vi "testConfig.vi"(8 "error in (no error)":errorcluster) -> (0 "error out":errorcluster)   [LabVIEW 2018]
uses:
  src/Logger/Logger.lvclass
  src/Logger/Logger.lvclass/Logger.ctl
  <vilib>/addons/_JKI Toolkits/Caraya/classes/Assert/Assert Equal Value_Variant.vi
  <vilib>/addons/_JKI Toolkits/Caraya/classes/Assert/Assert True.vi
  <vilib>/addons/_JKI Toolkits/Caraya/classes/Test/Test.lvclass
  <vilib>/addons/_JKI Toolkits/Caraya/classes/Assert/Assert.lvclass
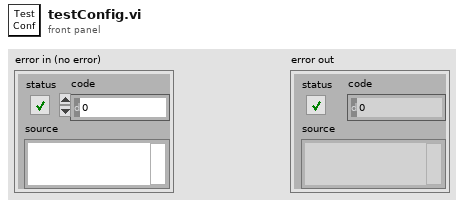
[diagram p1: front panel]
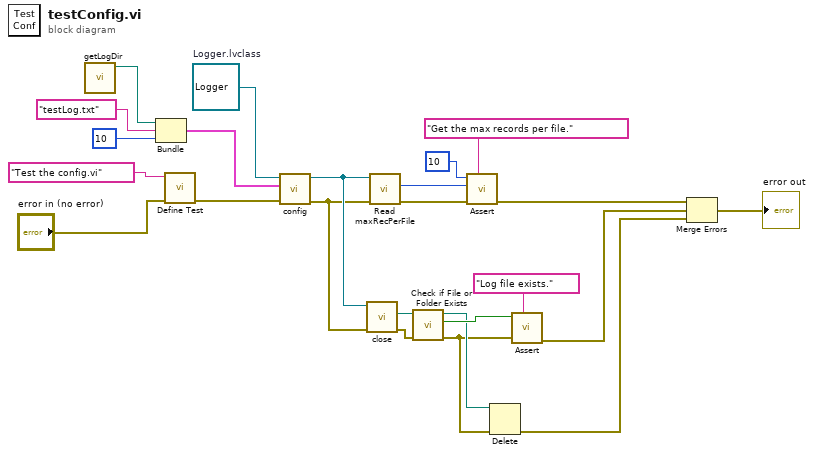
[diagram p0: block diagram]
diagram:
  w21 = refnum<class "Logger.lvclass"> refnum  # Logger.lvclass
  n1 = call "getLogDir.vi"() -> ("dirLog"=w20:path)  [unwired: 11 in]
  n2 = Bundle("dirLog"=w20, "testLog.txt", u32 10) -> (w17:cluster{"dirLog":path, string, u32})  [unwired: 1 in]
  n3 = call <vilib>:"Define Test.vi"("error in (no error)"="error in (no error)", "Label (VI Title)"="Test the config.vi") -> ("error out"=w22:errorcluster)  [unwired: 9 in]
  n4 = call "config.vi"("error in (no error)"=w22, "confData"=w17, "Logger in"=w21) -> ("error out"=w15:errorcluster, "Logger out"=w16:refnum<class "Logger.lvclass">)  [unwired: 7 in]
  n5 = call "close.vi"("error in (no error)"=w15, "Logger in"=w16) -> ("error out"=w9:errorcluster, "filePathClosed"=w10:path)  [unwired: 7 in, 1 out]
  n6 = call "Read maxRecPerFile.vi"("error in (no error)"=w15, "Logger in"=w16) -> ("error out"=w14:errorcluster, "maxRecPerFile"=w13:u32)  [unwired: 7 in, 1 out]
  n7 = call <vilib>:"Check if File or Folder Exists.vi"("error in (no error)"=w9, "path"=w10) -> ("error out"=w2:errorcluster, "file or folder exists?"=w8:bool, "dup path"=w3:path)  [unwired: 7 in]
  n8 = call-poly <vilib>:"Assert.vi"("Label"="Get the max records per file.", "error in (no error)"=w14, "Y"=w13, "X"=10) -> ("error out"=w6:errorcluster)  [unwired: 7 in]
  n9 = Delete(path (use dialog)=w3, error in=w2) -> (error out=w1:errorcluster)  [unwired: 3 in, 2 out]
  n10 = call-poly <vilib>:"Assert.vi"("Label"="Log file exists.", "error in (no error)"=w2, "True?"=w8) -> ("error out"=w5:errorcluster)  [unwired: 8 in]
  n11 = Merge Errors(w6, w5, w1) -> (→"error out":errorcluster)
